vi "Pre-Build VI - Run Unit Tests.vi"(8 "error in (no error)":errorcluster) -> (0 "error out":errorcluster, 1 "VIs without test coverage":string[](array[string]), 2 "error type":enum16{"fatal", "non-fatal", "warning"}(ring), 4 "VIs not loadable":string[](array[string]))   [LabVIEW 2020]
panel:
  out "VIs Failed":string[](array[string])
  out "VIs Succeeded":string[](array[string])
  in  "type specifier VI Refnum (for type only)":refnum<vi>
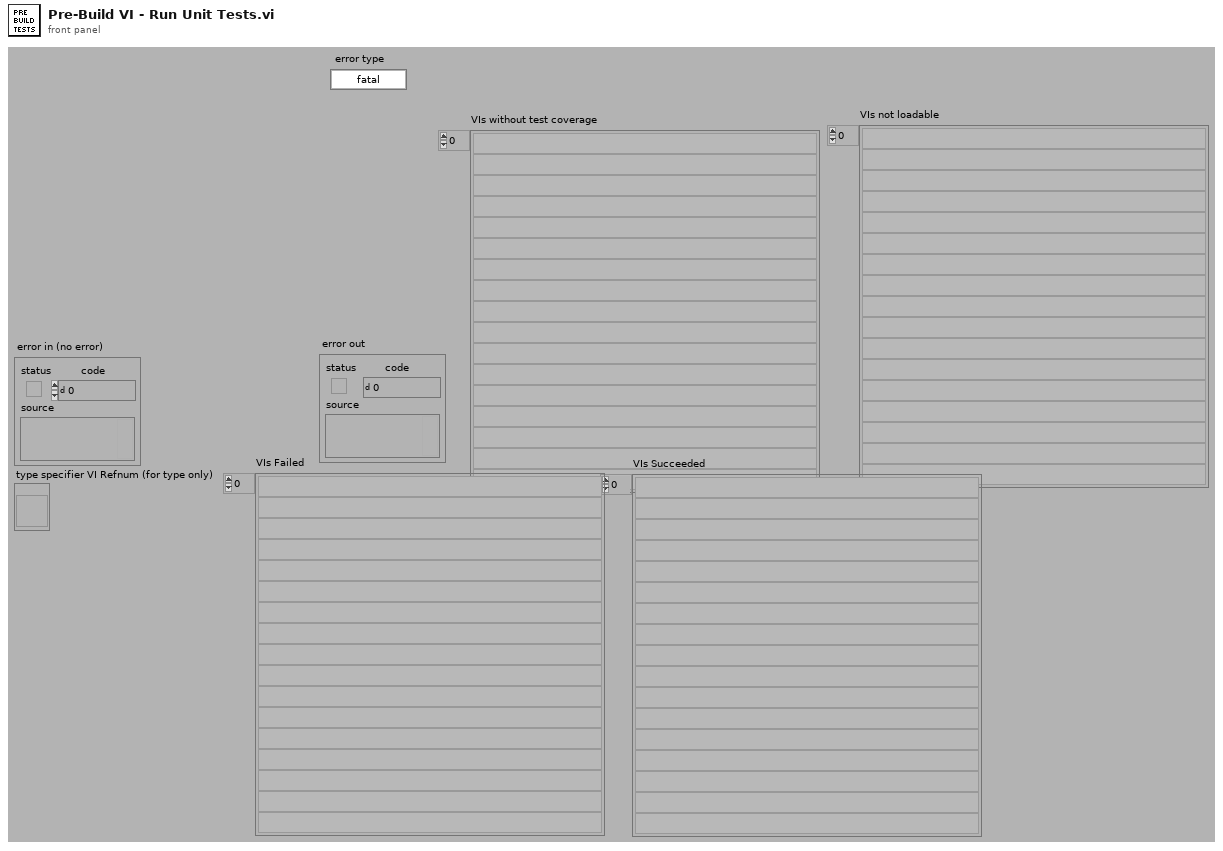
[diagram p1: front panel]
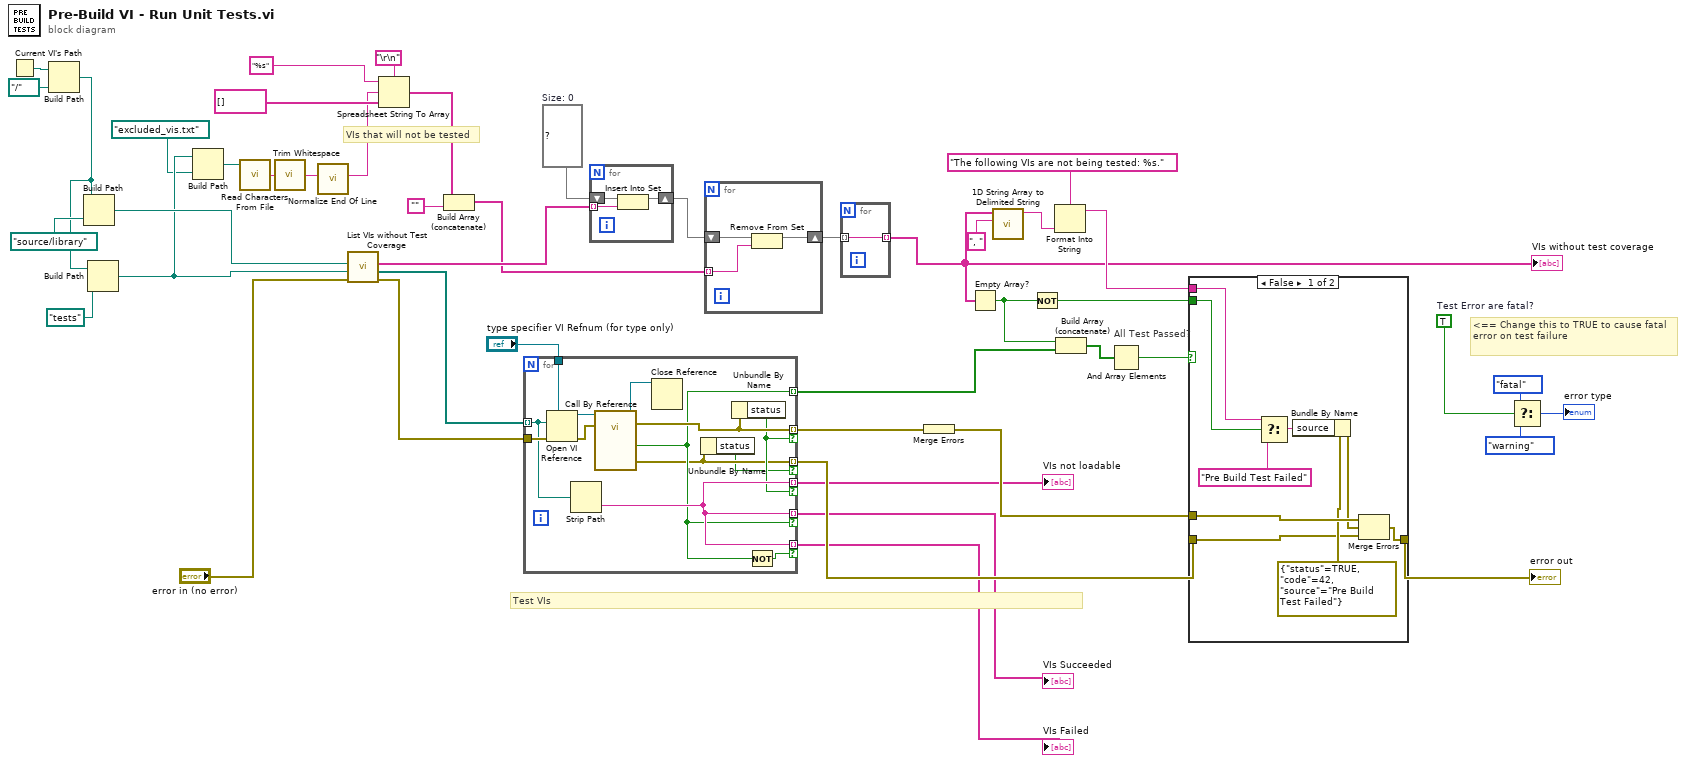
[diagram p0: block diagram]
diagram:
  w13 = set{string} {}  # Size: 0
  w37 = TRUE  # Test Error are fatal?
  # "VIs that will not be tested"
  # "<== Change this to TRUE to cause fatal error on test failure"
  # "All Test Passed?"
  # "Test VIs"
  n1 = Current VI's Path() -> (path=w22:path)
  n2 = Build Path(base path=w22, name or relative path=path "../..") -> (appended path=w18:path)
  n3 = Build Path(base path=w18, name or relative path=path "source/library" ("Relative path (.)")) -> (appended path=w20:path)
  n4 = Build Path(base path=w18, name or relative path=path "tests" ("Relative path (.)")) -> (appended path=w16:path)
  n5 = Build Path(base path=w16, name or relative path=path "excluded_vis.txt" ("Relative path (.)")) -> (appended path=w14:path)
  n6 = call <vilib>:"Read Characters From File.vi"("file path (dialog if empty)"=w14) -> ("character string"=w4:string)  [unwired: 5 in, 3 out]
  n7 = call <vilib>:"Trim Whitespace.vi"("string"=w4) -> ("trimmed string"=w2:string)  [unwired: 1 in]
  n8 = call <vilib>:"Normalize End Of Line.vi"("string in"=w2) -> ("string out"=w1:string)  [unwired: 7 in]
  n9 = call "List VIs without Test Coverage.vi"("error in (no error)"="error in (no error)", "Tests Root"=w16, "Source Root"=w20) -> ("error out"=w29:errorcluster, "Test VIs"=w33:path[], "VIs without test coverage"=w12:string[])  [unwired: 6 in]
  n10 = Spreadsheet String To Array(delimiter (Tab)="\r\n", format string="%s", spreadsheet string=w1, array type (2D Dbl)=string[] [] ("appended array")) -> (array=w3:string[])
  n11 = Build Array (concatenate)(w3, "") -> (w10:string[])
  n12 = for {
    tunnel: w33 -> [w54] mode=indexing
    tunnel: "type specifier VI Refnum (for type only)" -> [w60]
    tunnel: [w52] -> w26 mode=indexing
    tunnel: [w49] -> w31 mode=indexing if=w48
    tunnel: w29 -> [w56]
    tunnel: [w55] -> w27 mode=indexing if=w50
    tunnel: [w53] -> w25 mode=indexing if=w50
    tunnel: [w53] -> w24 mode=indexing if=w52
    tunnel: [w53] -> w23 mode=indexing if=w51
    n13 = Open VI Reference(type specifier VI Refnum (for type only)=w60, vi path=w54, error in (no error)=w56) -> (vi reference=w59:refnum<vi>, error out=w58:errorcluster)  [unwired: 3 in]
    n14 = Strip Path(path=w54) -> (name=w53:string)  [unwired: 1 out]
    n15 = call-by-ref "?"(reference=w59, error in=w58) -> (reference out=w57:refnum<vi>, error out=w55:errorcluster, 0:"error out"=w49:errorcluster, "pass"=w52:bool)  [unwired: 10 in]
    n16 = Close Reference(reference=w57) -> ()  [unwired: 1 in, 1 out]
    n17 = Unbundle By Name(w49) -> ("status"=w48:bool)
    n18 = Unbundle By Name(w55) -> ("status"=w50:bool)
    n19 = Not(x=w52) -> (.not. x?=w51:bool)
  }
  "VIs not loadable" <- w25
  "VIs Succeeded" <- w24
  "VIs Failed" <- w23
  n20 = for {
    tunnel: w12 -> [w63] mode=indexing
    shift-right: [w61] -> w11
    shift-left: w13 -> [w62]
    n21 = Insert Into Set(10:w63, 11:w62) -> (3:w61:set{string})  [unwired: 1 out]
  }
  n22 = for {
    shift-right: [w64] -> w9
    shift-left: w11 -> [w66]
    tunnel: w10 -> [w65] mode=indexing
    n23 = Remove From Set(10:w65, 11:w66) -> (3:w64:set{string})  [unwired: 1 out]
  }
  n24 = for {
    tunnel: [w67] -> w8 mode=indexing
    tunnel: w9 -> [w67] mode=indexing
  }
  "VIs without test coverage" <- w8
  n25 = Merge Errors(w27) -> (w28:errorcluster)
  n26 = Empty Array?(array=w8) -> (empty?=w41:bool)
  n27 = call <vilib>:"1D String Array to Delimited String.vi"("delimiter"=", " ("delimiter (Tab)"), "string array"=w8) -> ("delimited string"=w44:string)  [unwired: 9 in]
  n28 = Not(x=w41) -> (.not. x?=w40:bool)
  n29 = Format Into String(format string="The following VIs are not being tested: %s.", w44) -> (resulting string=w42:string)  [unwired: 2 in, 1 out]
  n30 = Build Array (concatenate)(w41, w26) -> (w47:bool[])
  n31 = And Array Elements(Boolean array=w47) -> (logical AND=w46:bool)
  n32 = case shown="False" w46 {
    tunnel: w28 -> [w76 w77]
    tunnel: [w75 w77] -> w39
    tunnel: w40 -> [w74 _]
    tunnel: w42 -> [w73 _]
    tunnel: w31 -> [w68 _]
    frame False {
      n33 = Select(t=w73, s=w74, f="Pre Build Test Failed" ("source")) -> (s? t:f=w71:string)
      n34 = Bundle By Name(cluster=errorcluster {"status"=TRUE, "code"=42, "source"="Pre Build Test Failed"} ("error out"), "source"=w71) -> (w70:errorcluster)
      n35 = Merge Errors(w76, w70, w68) -> (w75:errorcluster)
    }
    frame True {
    }
  }
  "error out" <- w39
  n36 = Select(t=enum16{"fatal", "non-fatal", "warning"}."fatal" ("error type"), s=w37, f=enum16{"fatal", "non-fatal", "warning"}."warning" ("error type")) -> (s? t:f=→"error type":enum16{"fatal", "non-fatal", "warning"})
